vi "Stop Core.vi"(10 "final error code":i32, 11 "Measure Object in":refnum<class "Pulse Controller.lvclass">) -> (3 "Measure Object out":refnum<class "Pulse Controller.lvclass">)   [LabVIEW 2024, in "Pulse Controller.lvclass"]
doc: "(<B>Filename</B>: Actor Framework.lvlib:Actor.lvclass:Stop Core.vi)\n\nDefines what the actor does before it stops. Use the <B>final error code</B> input to determine whether the actor shut down in response to an error.\n\nBy default, this method does nothing. A descendant class may override it to define behavior, such as shutting down any processes the actor initiated in its override of the Actor Core method."
uses:
  Pulse Controller.lvclass
  Pulse Controller.lvclass/Pulse Controller.ctl
  Process Controller/Process Controller.lvclass
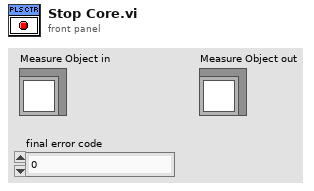
[diagram p1: front panel]
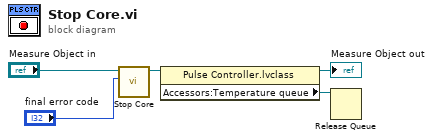
[diagram p0: block diagram]
diagram:
  n1 = call-parent "Stop Core.vi"("final error code"="final error code", "Measure Object in"="Measure Object in") -> ("Measure Object out"=w5:refnum<class "Pulse Controller.lvclass">)  [unwired: 9 in]
  n2 = property class="Pulse Controller.lvclass"(reference=w5) -> (reference out=→"Measure Object out":refnum<class "Pulse Controller.lvclass">, "Accessors:Temperature queue"=w1:refnum<queue>)  [unwired: 1 in, 1 out]
  n3 = Release Queue(queue=w1) -> ()  [unwired: 2 in, 3 out]
